vi "ConfigFiles_Write&Read.vi"(5 "功能类型":enum16{"读取", "写入"}(ring), 6 "error in (no error)":errorcluster caption="错误输入（无错误）", 7 "configuration file path":path caption="配置文件的路径", 8 "键值_输入":variant=variant(string "4"), 9 "键值类型":T1(ring), 10 "键名称":string, 11 "字段名称":string) -> (1 "键值_输出":variant, 2 "找到?":bool, 3 "file path":path caption="文件路径", 4 "error out":errorcluster caption="错误输出")   [LabVIEW 2018]
uses:
  <vilib>/Utility/config.llb/Read Key (Boolean).vi
  <vilib>/Utility/config.llb/Read Key (Double).vi
  <vilib>/Utility/config.llb/Read Key (I32).vi
  <vilib>/Utility/config.llb/Read Key (Path).vi
  <vilib>/Utility/config.llb/Read Key (String).vi
  <vilib>/Utility/config.llb/Read Key (U32).vi
  <vilib>/Utility/config.llb/Write Key (Boolean).vi
  <vilib>/Utility/config.llb/Write Key (Double).vi
  <vilib>/Utility/config.llb/Write Key (I32).vi
  <vilib>/Utility/config.llb/Write Key (Path).vi
  <vilib>/Utility/config.llb/Write Key (String).vi
  <vilib>/Utility/config.llb/Write Key (U32).vi
  <vilib>/Utility/config.llb/NI_LVConfig.lvlib
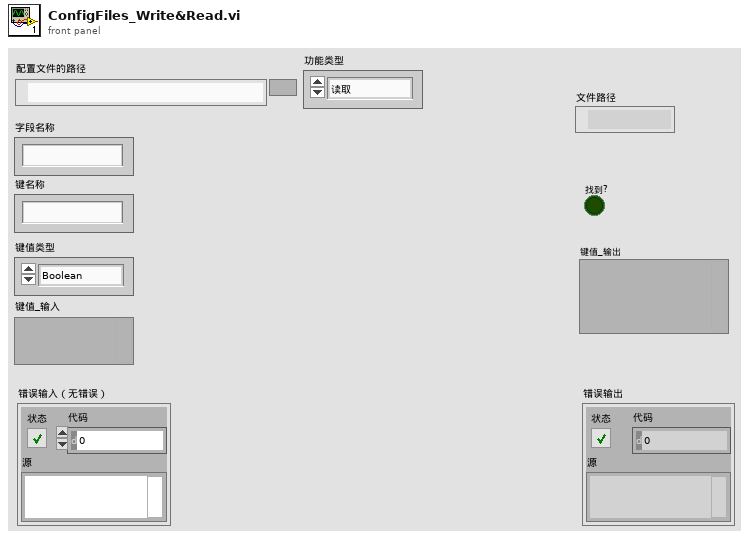
[diagram p1: front panel]
types:
  T1 = enum16{"Boolean", "DBL", "I32", "Path", "String", "U32"}
  T2 = typedef "NI_LVConfig.lvlib/Config Data RefNum.ctl" = refnum<k1>
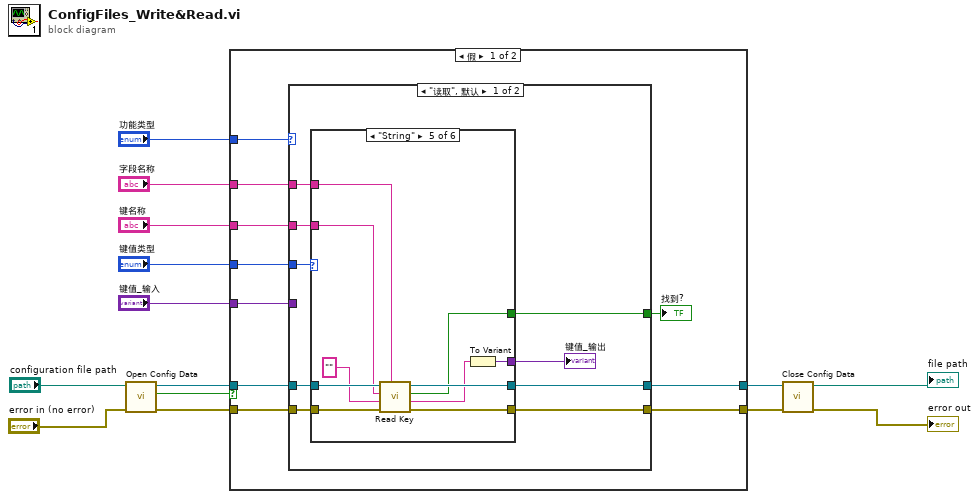
[diagram p0: block diagram]
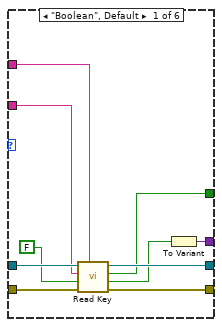
[diagram p2: hidden frame]
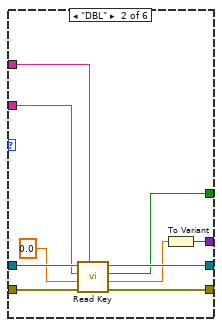
[diagram p3: hidden frame]
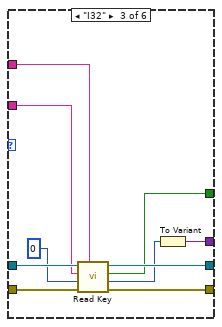
[diagram p4: hidden frame]
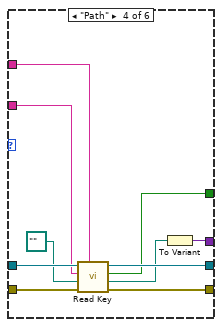
[diagram p5: hidden frame]
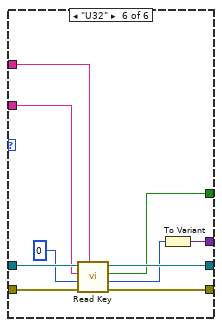
[diagram p6: hidden frame]
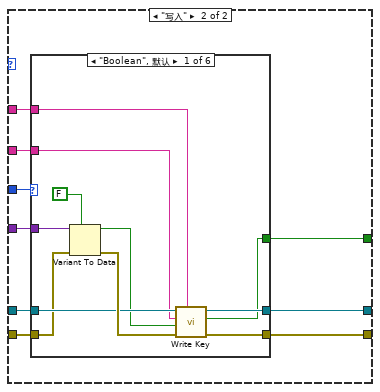
[diagram p7: hidden frame]
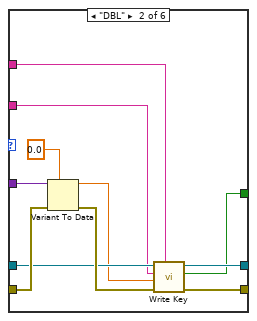
[diagram p8: hidden frame]
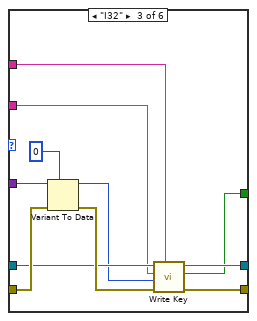
[diagram p9: hidden frame]
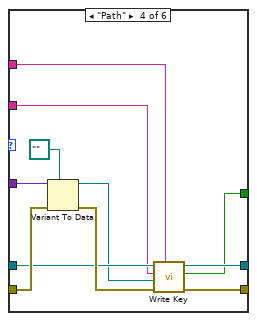
[diagram p10: hidden frame]
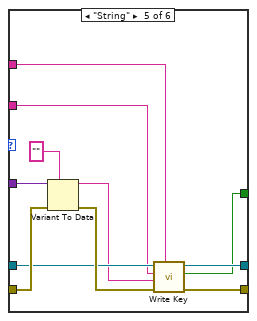
[diagram p11: hidden frame]
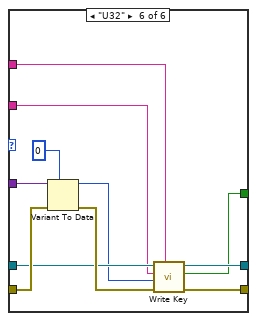
[diagram p12: hidden frame]
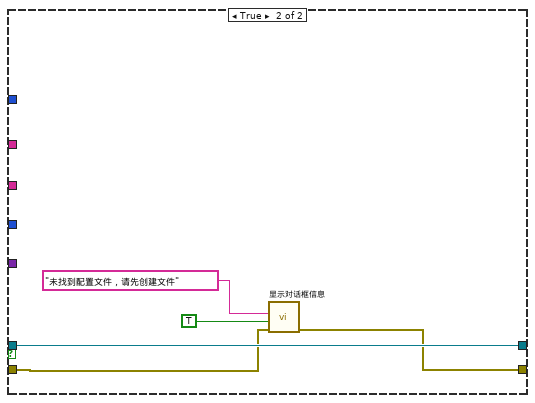
[diagram p13: hidden frame]
diagram:
  n1 = call <vilib>:"Open Config Data.vi"("error in (no error)"="error in (no error)", "configuration file path"="configuration file path") -> ("error out"=w11:errorcluster, "file created?"=w2:bool, "refnum"=w12:T2)  [unwired: 7 in]
  n2 = case shown="假" w2 {
    tunnel: w12 -> [w24 w173]
    tunnel: w11 -> [w23 w172]
    tunnel: [w22 w173] -> w10
    tunnel: [w21 w171] -> w9
    tunnel: "功能类型" -> [w20 _]
    tunnel: "字段名称" -> [w19 _]
    tunnel: "键值_输入" -> [w18 _]
    tunnel: "键值类型" -> [w17 _]
    tunnel: "键名称" -> [w16 _]
    frame False {
      n3 = case shown="\"读取\", 默认" w20 {
        tunnel: w24 -> [w33 w98]
        tunnel: w23 -> [w32 w102]
        tunnel: [w31 w99] -> w22
        tunnel: [w30 w95] -> w21
        tunnel: w19 -> [w27 w97]
        tunnel: w18 -> [_ w101]
        tunnel: w17 -> [w29 w100]
        tunnel: w16 -> [w28 w96]
        tunnel: [w25 w94] -> w15
        frame "读取", Default {
          n4 = case shown="\"String\"" w29 {
            tunnel: w32 -> [w38 w48 w58 w68 w78 w88]
            tunnel: [w43 w53 w63 w73 w83 w93] -> w30
            tunnel: [w42 w52 w62 w72 w82 w92] -> w31
            tunnel: w33 -> [w41 w51 w61 w71 w81 w91]
            tunnel: w27 -> [w40 w50 w60 w70 w80 w90]
            tunnel: w28 -> [w39 w49 w59 w69 w79 w89]
            tunnel: [w35 w46 w56 w66 w76 w86] -> w26
            tunnel: [w34 w44 w54 w64 w74 w84] -> w25
            frame "Boolean", Default {
              n5 = call-poly <vilib>:"Read Key.vi"("section"=w40, "error in (no error)"=w38, "default value"=FALSE, "key"=w39, "refnum"=w41) -> ("error out"=w43:errorcluster, "value"=w36:bool, "found?"=w34:bool, "refnum out"=w42:T2)  [unwired: 3 in]
              n6 = To Variant(anything=w36) -> (Variant=w35:variant)
            }
            frame "DBL" {
              n7 = call-poly <vilib>:"Read Key.vi"("section"=w50, "error in (no error)"=w48, "default value"=0.0, "key"=w49, "refnum"=w51) -> ("error out"=w53:errorcluster, "value"=w45:dbl, "found?"=w44:bool, "refnum out"=w52:T2)  [unwired: 3 in]
              n8 = To Variant(anything=w45) -> (Variant=w46:variant)
            }
            frame "I32" {
              n9 = call-poly <vilib>:"Read Key.vi"("section"=w60, "error in (no error)"=w58, "default value"=0, "key"=w59, "refnum"=w61) -> ("error out"=w63:errorcluster, "value"=w55:i32, "found?"=w54:bool, "refnum out"=w62:T2)  [unwired: 3 in]
              n10 = To Variant(anything=w55) -> (Variant=w56:variant)
            }
            frame "Path" {
              n11 = call-poly <vilib>:"Read Key.vi"("section"=w70, "error in (no error)"=w68, "default value"=path "" ("configuration file path"), "key"=w69, "refnum"=w71) -> ("error out"=w73:errorcluster, "value"=w65:path, "found?"=w64:bool, "refnum out"=w72:T2)  [unwired: 3 in]
              n12 = To Variant(anything=w65) -> (Variant=w66:variant)
            }
            frame "String" {
              n13 = call-poly <vilib>:"Read Key.vi"("section"=w80, "error in (no error)"=w78, "default value"="", "key"=w79, "refnum"=w81) -> ("error out"=w83:errorcluster, "value"=w75:string, "found?"=w74:bool, "refnum out"=w82:T2)  [unwired: 3 in]
              n14 = To Variant(anything=w75) -> (Variant=w76:variant)
            }
            frame "U32" {
              n15 = call-poly <vilib>:"Read Key.vi"("section"=w90, "error in (no error)"=w88, "default value"=u32 0, "key"=w89, "refnum"=w91) -> ("error out"=w93:errorcluster, "value"=w85:u32, "found?"=w84:bool, "refnum out"=w92:T2)  [unwired: 3 in]
              n16 = To Variant(anything=w85) -> (Variant=w86:variant)
            }
          }
          "键值_输出" <- w26
        }
        frame "写入" {
          n17 = case shown="\"Boolean\", 默认" w100 {
            tunnel: w102 -> [w104 w123 w134 w145 w156 w167]
            tunnel: [w110 w121 w132 w143 w154 w165] -> w95
            tunnel: w101 -> [w113 w124 w135 w146 w157 w168]
            tunnel: [w109 w120 w131 w142 w153 w164] -> w99
            tunnel: w98 -> [w108 w119 w130 w141 w152 w163]
            tunnel: w97 -> [w106 w117 w128 w139 w150 w161]
            tunnel: w96 -> [w105 w116 w127 w138 w149 w160]
            tunnel: [w103 w114 w125 w136 w147 w158] -> w94
            frame "Boolean", Default {
              n18 = Variant To Data(error in=w104, type=FALSE, Variant=w113) -> (data=w107:bool, error out=w111:errorcluster)
              n19 = call-poly <vilib>:"Write Key.vi"("section"=w106, "error in (no error)"=w111, "value"=w107, "key"=w105, "refnum"=w108) -> ("error out"=w110:errorcluster, "found?"=w103:bool, "refnum out"=w109:T2)  [unwired: 4 in]
            }
            frame "DBL" {
              n20 = Variant To Data(error in=w123, type=0.0, Variant=w124) -> (data=w118:dbl, error out=w122:errorcluster)
              n21 = call-poly <vilib>:"Write Key.vi"("section"=w117, "error in (no error)"=w122, "value"=w118, "key"=w116, "refnum"=w119) -> ("error out"=w121:errorcluster, "found?"=w114:bool, "refnum out"=w120:T2)  [unwired: 4 in]
            }
            frame "I32" {
              n22 = Variant To Data(error in=w134, type=0, Variant=w135) -> (data=w129:i32, error out=w133:errorcluster)
              n23 = call-poly <vilib>:"Write Key.vi"("section"=w128, "error in (no error)"=w133, "value"=w129, "key"=w127, "refnum"=w130) -> ("error out"=w132:errorcluster, "found?"=w125:bool, "refnum out"=w131:T2)  [unwired: 4 in]
            }
            frame "Path" {
              n24 = Variant To Data(error in=w145, type=path "" ("configuration file path"), Variant=w146) -> (data=w140:path, error out=w144:errorcluster)
              n25 = call-poly <vilib>:"Write Key.vi"("section"=w139, "error in (no error)"=w144, "value"=w140, "key"=w138, "refnum"=w141) -> ("error out"=w143:errorcluster, "found?"=w136:bool, "refnum out"=w142:T2)  [unwired: 4 in]
            }
            frame "String" {
              n26 = Variant To Data(error in=w156, type="", Variant=w157) -> (data=w151:string, error out=w155:errorcluster)
              n27 = call-poly <vilib>:"Write Key.vi"("section"=w150, "error in (no error)"=w155, "value"=w151, "key"=w149, "refnum"=w152) -> ("error out"=w154:errorcluster, "found?"=w147:bool, "refnum out"=w153:T2)  [unwired: 4 in]
            }
            frame "U32" {
              n28 = Variant To Data(error in=w167, type=u32 0, Variant=w168) -> (data=w162:u32, error out=w166:errorcluster)
              n29 = call-poly <vilib>:"Write Key.vi"("section"=w161, "error in (no error)"=w166, "value"=w162, "key"=w160, "refnum"=w163) -> ("error out"=w165:errorcluster, "found?"=w158:bool, "refnum out"=w164:T2)  [unwired: 4 in]
            }
          }
        }
      }
      "找到?" <- w15
    }
    frame True {
      n30 = call "显示对话框信息"("error in (no error)"=w172, "Enable"=TRUE, "Message"="未找到配置文件，请先创建文件") -> ("error out"=w171:errorcluster)  [unwired: 7 in, 1 out]
    }
  }
  n31 = call <vilib>:"Close Config Data.vi"("error in (no error)"=w9, "refnum"=w10) -> ("error out"=→"error out":errorcluster, "file path"=→"file path":path)  [unwired: 8 in]
